vi "Button Toggle.vi"(5 "Button Input":bool) -> (2 "Toggled Output":bool)   [LabVIEW 2013]
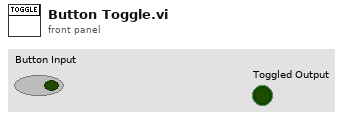
[diagram p1: front panel]
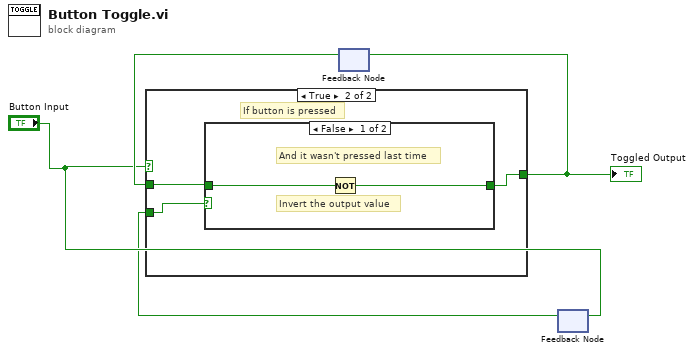
[diagram p0: block diagram]
diagram:
  n1 = feedback #1() -> (w4:bool)  [unwired: 1 in]
  n2 = feedback-in #2("Button Input") -> ()
  n3 = feedback #2() -> (w2:bool)  [unwired: 1 in]
  n4 = case shown="True" "Button Input" {
    tunnel: w4 -> [w5 w8]
    tunnel: [w5 w7] -> w1
    tunnel: w2 -> [_ w6]
    frame False {
      # "Use previous value"
      # "Button not pressed"
    }
    frame True {
      # "If button is pressed"
      n5 = case shown="False" w6 {
        tunnel: w8 -> [w10 w11]
        tunnel: [w9 w11] -> w7
        frame False {
          # "Invert the output value"
          # "And it wasn't pressed last time"
          n6 = Not(x=w10) -> (.not. x?=w9:bool)
        }
        frame True {
          # "Keep the previous value"
          # "And it was pressed last time"
        }
      }
    }
  }
  "Toggled Output" <- w1
  n7 = feedback-in #1(w1) -> ()
